vi "Temperature Limit.vi"() -> ()   [LabVIEW 2015]
doc: "This VI simulates the acquisition of temperature, graphs the temperature, and notifies the user if the temperature is over the limit."
panel:
  in  "Start":bool
  in  "Delta t (ms)":i32(slide)=400 scale=50.0..500.0
  in  "Stop":bool
  in  "High Limit":dbl=28.0 format="%.2f"
  out "Temperature":cluster{"Temperature":dbl, "High Limit":dbl}(graph)={"Temperature"=85.88749999999999, "High Limit"=80.0}
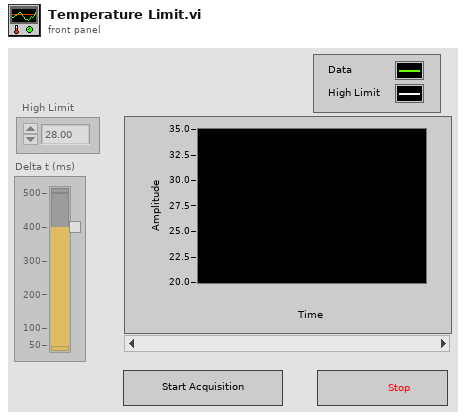
[diagram p1: front panel]
types:
  T1 = enum8{"Enabled", "Disabled", "Disabled and Grayed Out"}
  T2 = cluster{"Temperature Value":dbl, "High Limit":dbl}
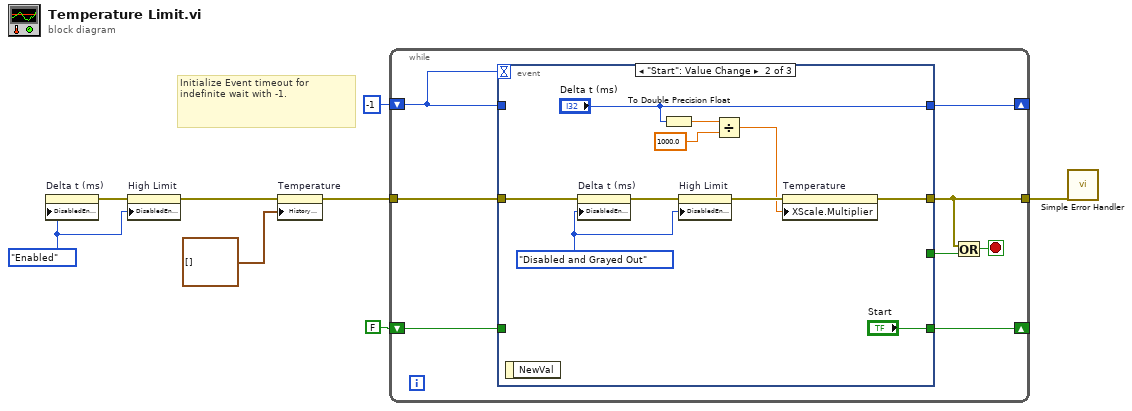
[diagram p0: block diagram]
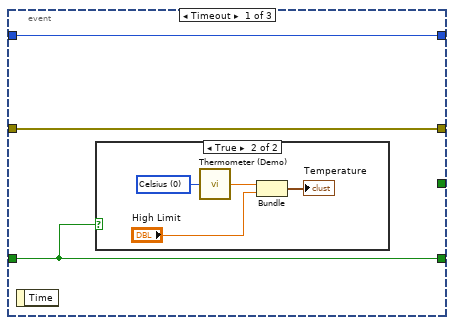
[diagram p2: hidden frame]
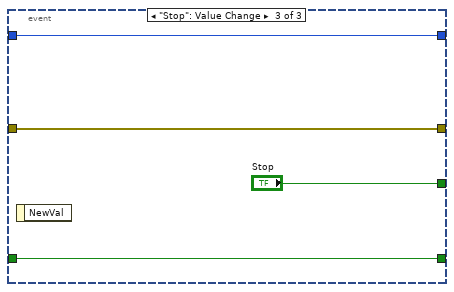
[diagram p4: hidden frame]
diagram:
  w4 = T1."Enabled" ("Disabled")
  # "Initialize Event timeout for indefinite wait with -1."
  n1 = property on="Delta t (ms)" class="Slide (strict)"("DisabledEnum"=w4) -> (error out=w5:errorcluster)  [unwired: 2 in, 1 out]
  n2 = property on="High Limit" class="DigNum (strict)"(error in=w5, "DisabledEnum"=w4) -> (error out=w2:errorcluster)  [unwired: 1 in, 1 out]
  n3 = property on="Temperature" class="WFChart (strict)"(error in=w2, "History Data"=cluster{"Temperature":dbl, "High Limit":dbl}[] []) -> (error out=w3:errorcluster)  [unwired: 1 in, 1 out]
  n4 = while {
    tunnel: w3 -> [w16]
    tunnel: [w14] -> w7
    shift-right: [w12] -> _
    shift-left: FALSE ("Start") -> [w11]
    shift-right: [w10] -> _
    shift-left: -1 ("Delta t (ms)") -> [w9]
    stop <- w15 stop-if-true
    n5 = event shown="[1] \"Start\": Value Change" {
      selector: _ -> [_ _ _]
      dyn-events: _ -> [_ _ _]
      timeout: w9 -> [_ _ _]
      tunnel: [_ _ "Stop"] -> w13
      tunnel: w16 -> [w19 w32 w36]
      tunnel: [w19 w28 w36] -> w14
      tunnel: [w17 "Start" w35] -> w12
      tunnel: w11 -> [w17 _ w35]
      tunnel: [w18 "Delta t (ms)" w34] -> w10
      tunnel: w9 -> [w18 _ w34]
      event Timeout {
        n6 = event-data() -> ()  [unwired: 1 in, 1 out]
        n7 = case shown="True" w17 {
          frame False {
          }
          frame True {
            w20 = u16 0 items=["Celsius", "Fahrenheit"] ("Units (0: Celsius)")
            n8 = call "Thermometer (Demo).vi"("Units (0: Celsius)"=w20) -> ("Temperature Value"=w21:dbl)
            n9 = Bundle("Temperature Value"=w21, "High Limit"="High Limit") -> (→"Temperature":T2)  [unwired: 1 in]
          }
        }
      }
      event "Start": Value Change {
        w30 = T1."Disabled and Grayed Out" ("Disabled")
        n10 = event-data() -> ()  [unwired: 1 in, 1 out]
        n11 = property on="Delta t (ms)" class="Slide (strict)"(error in=w32, "DisabledEnum"=w30) -> (error out=w31:errorcluster)  [unwired: 1 in, 1 out]
        n12 = To Double Precision Float(number="Delta t (ms)") -> (double precision float=w26:dbl)
        n13 = property on="High Limit" class="DigNum (strict)"(error in=w31, "DisabledEnum"=w30) -> (error out=w29:errorcluster)  [unwired: 1 in, 1 out]
        n14 = Divide(x=w26, y=1000.0) -> (x/y=w24:dbl)
        n15 = property on="Temperature" class="WFChart (strict)"(error in=w29, "XScale.Multiplier"=w24) -> (error out=w28:errorcluster)  [unwired: 1 in, 1 out]
      }
      event "Stop": Value Change {
        n16 = event-data() -> ()  [unwired: 1 in, 1 out]
      }
    }
    n17 = Or(x=w14, y=w13) -> (x .or. y?=w15:bool)
  }
  n18 = call <vilib>:"Simple Error Handler.vi"("error in (no error)"=w7) -> ()  [unwired: 4 in, 5 out]
